vi "Component Comparator.vi"(1 "Input 2":T1, 2 "Input 1":T1) -> (0 "Output":bool)   [LabVIEW 2020]
uses:
  Component.ctl
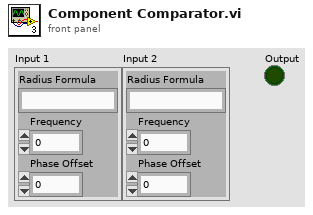
[diagram p1: front panel]
types:
  T1 = typedef "Component.ctl" = cluster{"Radius Formula":string, "Frequency":dbl, "Phase Offset":dbl}
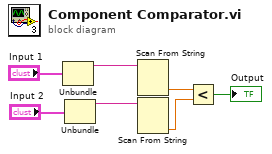
[diagram p0: block diagram]
diagram:
  n1 = Unbundle("Input 1") -> ("Radius Formula"=w5:string)  [unwired: 2 out]
  n2 = Unbundle("Input 2") -> ("Radius Formula"=w4:string)  [unwired: 2 out]
  n3 = Scan From String(input string=w5) -> (output 1=w3:dbl)  [unwired: 4 in, 3 out]
  n4 = Scan From String(input string=w4) -> (output 1=w2:dbl)  [unwired: 4 in, 3 out]
  n5 = Less?(x=w3, y=w2) -> (x < y?=→"Output":bool)
